vi "Z-Scan-20.vi"() -> ()   [LabVIEW 2014]
doc: "André Romero - 2020\nandretec@ifsc.usp.br"
uses:
  Z-Temporal-Signal.ctl
  <vilib>/Analysis/NI_AALBase.lvlib
panel:
  out "standard deviation":dbl format="%0.6f"
  out "ti/tf mean":dbl format="%0.2f"
  out "ti/tf Signal":dbl(graph)
  out "Number of samples":i32=4
  out "Time between acquire (ms)":u32=218
  out "Signal":dbl[][](graph)
  in  "rate":dbl=50000.0
  in  "N Samples":i64=8000
  out "Process time":string
  in  "Start Acquire":bool
  in  "Stop Acquire":bool
  out "Z Scan":cluster{"X":dbl, "Y":dbl}[](graph)
  # "DAQ Settings"
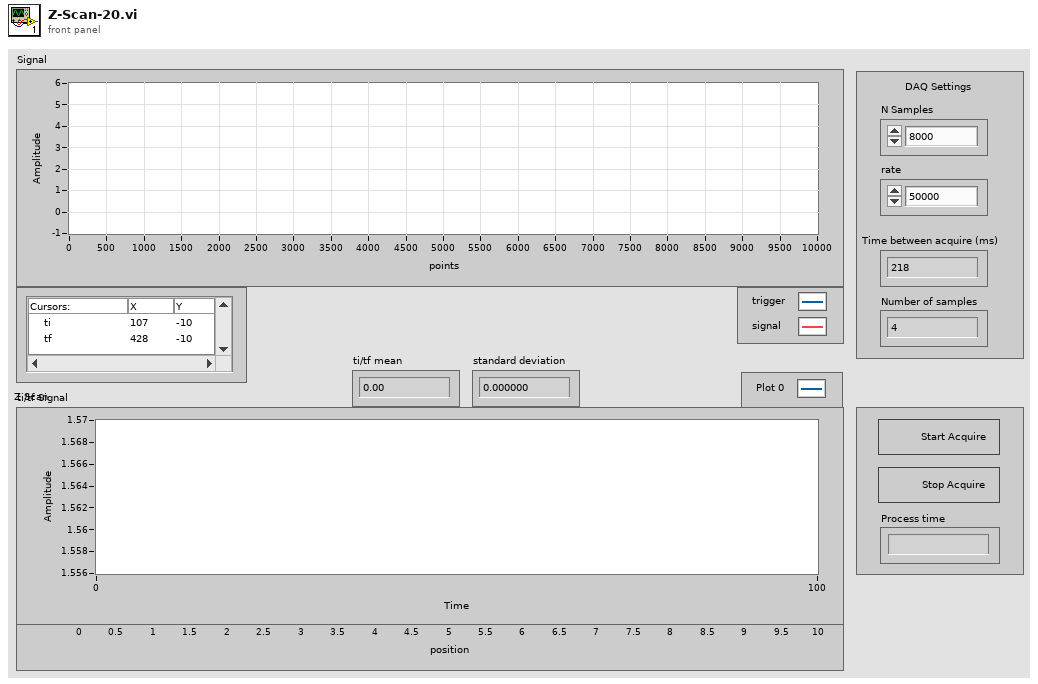
[diagram p1: front panel]
types:
  T1 = typedef "Z-Temporal-Signal.ctl" = cluster{"Signal State":string, "Signal":dbl[][], "ti":i32, "tf":i32, "Error":errorcluster}
  T2 = typedef "LVCursorListTypeDef.ctl" = cluster{"Name":string, "Color":u32, "Style":u8, "Point Style":u8, "Name Visible":bool, "Allow Drag":bool, "Cursor Mode":u32, "Plot":i32, "Index":i32, "Position":cluster{"X":dbl, "Y":dbl}, "X Scale":u32, "Y Scale":u32, "Watch Plots":i32[], "Watch All Plots":bool, "Plot Area":i32, "Label Offset":cluster{"X":dbl, "Y":dbl}}[]
  T3 = cluster{"Name":string, "Color":u32, "Style":u8, "Point Style":u8, "Name Visible":bool, "Allow Drag":bool, "Cursor Mode":u32, "Plot":i32, "Index":i32, "Position":cluster{"X":dbl, "Y":dbl}, "X Scale":u32, "Y Scale":u32, "Watch Plots":i32[], "Watch All Plots":bool, "Plot Area":i32, "Label Offset":cluster{"X":dbl, "Y":dbl}}
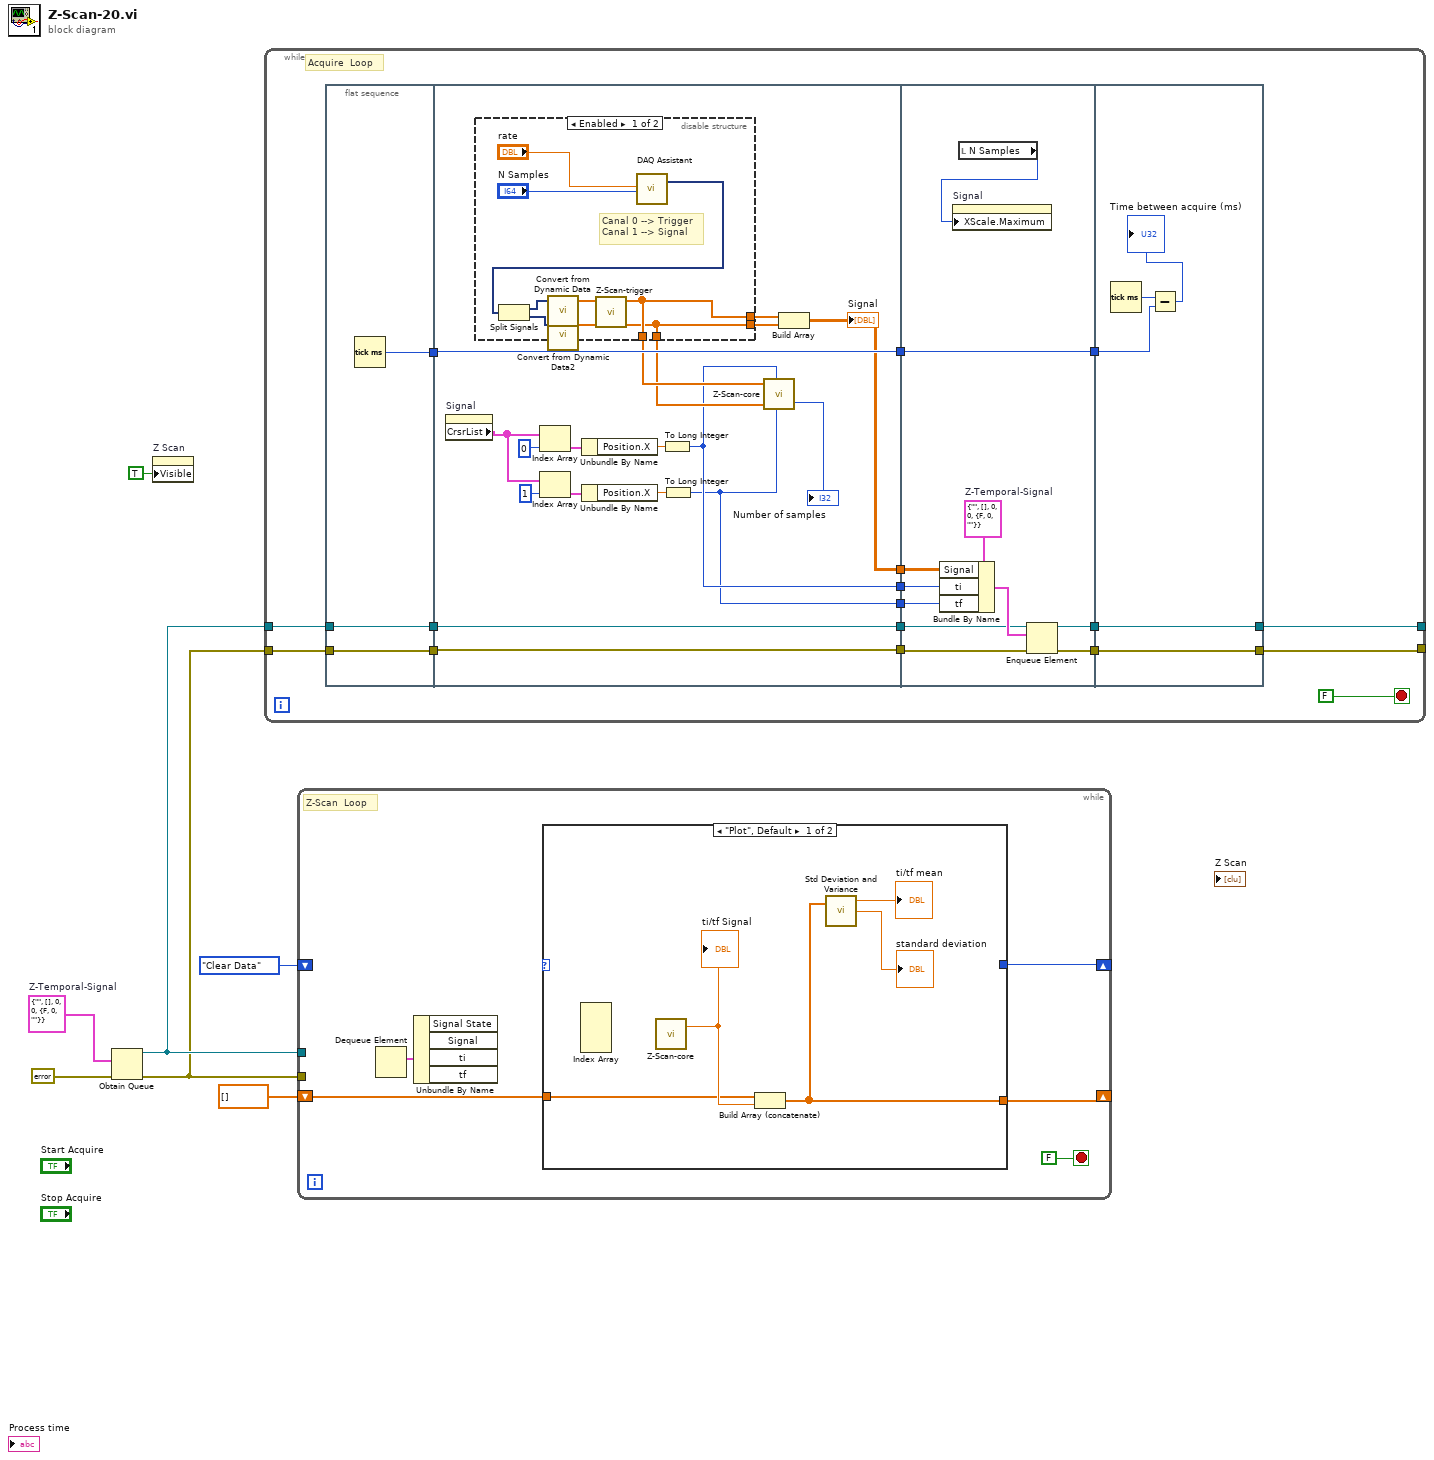
[diagram p0: block diagram]
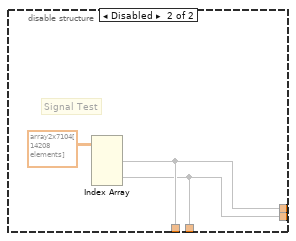
[diagram p2: hidden frame]
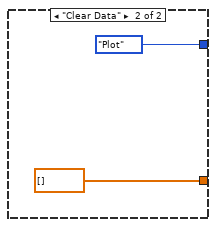
[diagram p3: hidden frame]
diagram:
  w4 = T1 {"Signal State"="", "Signal"=[], "ti"=0, "tf"=0, "Error"={"status"=FALSE, "code"=0, "source"=""}}  # Z-Temporal-Signal
  n1 = Obtain Queue(element data type=w4, error in (no error)=errorcluster {"status"=FALSE, "code"=0, "source"=""}) -> (queue out=w6:refnum<queue>, error out=w5:errorcluster)  [unwired: 3 in, 1 out]
  n2 = property on="Z Scan" class="XYGraph (strict)"("Visible"=TRUE) -> ()  [unwired: 2 in, 2 out]
  n3 = while {
    tunnel: w6 -> [w21]
    tunnel: w5 -> [w20]
    tunnel: [w18] -> _
    tunnel: [w8] -> _
    stop <- FALSE stop-if-true
    # "Acquire  Loop"
    n4 = flat-sequence {
      tunnel: [w27] -> w23
      tunnel: [w26] -> w22
      tunnel: w21 -> [w26]
      tunnel: w20 -> [w25]
      tunnel: [w25] -> w19
      tunnel: w23 -> [w43]
      tunnel: [w43] -> w17
      tunnel: w22 -> [w29]
      tunnel: w19 -> [w28]
      tunnel: [w32] -> w13
      tunnel: [w31] -> w12
      tunnel: [w30] -> w11
      tunnel: [w29] -> w10
      tunnel: [w28] -> w9
      tunnel: w17 -> [w68]
      tunnel: [w68] -> w16
      tunnel: [w65] -> w15
      tunnel: [w64] -> w14
      tunnel: w13 -> [w63]
      tunnel: w12 -> [w62]
      tunnel: w11 -> [w61]
      tunnel: w10 -> [w60]
      tunnel: w9 -> [w59]
      tunnel: w16 -> [w72]
      tunnel: [w70] -> w18
      tunnel: w15 -> [w70]
      tunnel: w14 -> [w69]
      tunnel: [w69] -> w8
      frame #0 {
        n5 = Tick Count (ms)() -> (millisecond timer value=w27:u32)
      }
      frame #1 {
        n6 = property on="Signal" class="WFGraph (strict)"() -> ("CrsrList"=w35:T2)  [unwired: 2 in, 2 out]
        n7 = disable-structure shown="Enabled" {
          disable-tunnel: [w47 w56] -> w45
          disable-tunnel: [w46 w55] -> w44
          disable-tunnel: [w47 w56] -> w34
          disable-tunnel: [w46 w55] -> w33
          frame Enabled {
            # "Canal 0 --> Trigger\nCanal 1 --> Signal"
            n8 = call "DAQ Assistant"("rate"="rate", "number of samples"="N Samples") -> ("data"=w52:dynamicdata)  [unwired: 15 in, 2 out]
            n9 = Split Signals(w52) -> (w51:dynamicdata, w50:dynamicdata)  [unwired: 2 in]
            n10 = call "Convert from Dynamic Data"("Dynamic Data Type"=w51) -> ("Array"=w49:dbl[])  [unwired: 3 in]
            n11 = call "Convert from Dynamic Data2"("Dynamic Data Type"=w50) -> ("Array"=w48:dbl[])  [unwired: 3 in]
            n12 = call "Z-Scan-trigger.vi"("signal in"=w48, "trigger in"=w49) -> ("signal out"=w46:dbl[], "trigger out"=w47:dbl[])  [unwired: 5 in, 1 out]
          }
          frame Disabled {
            # "Signal Test"
            n13 = Index Array(array=dbl[][] array2x7104[14208 elements] ("Signal 2")) -> (element #1=w56:dbl[], element #2=w55:dbl[])  [unwired: 4 in]
          }
        }
        n14 = Index Array(array=w35, index=0) -> (element=w38:T3)
        n15 = Index Array(array=w35, index=1) -> (element=w39:T3)
        n16 = Unbundle By Name(w38) -> ("Position.X"=w40:dbl)
        n17 = Unbundle By Name(w39) -> ("Position.X"=w41:dbl)
        n18 = To Long Integer(number=w40) -> (32bit integer=w31:i32)
        n19 = To Long Integer(number=w41) -> (32bit integer=w30:i32)
        n20 = call "Z-Scan-core.vi"("trigger in"=w34, "ti"=w31, "signal in"=w33, "tf"=w30) -> ("number of samples"=→"Number of samples":i32)  [unwired: 1 in, 1 out]
        n21 = Build Array(w45, w44) -> (w32:dbl[][])
        "Signal" <- w32
      }
      frame #2 {
        w67 = T1 {"Signal State"="", "Signal"=[], "ti"=0, "tf"=0, "Error"={"status"=FALSE, "code"=0, "source"=""}}  # Z-Temporal-Signal
        n22 = Bundle By Name(cluster=w67, "Signal"=w63, "ti"=w62, "tf"=w61) -> (w66:T1)
        n23 = local read "N Samples"() -> (w58:i64)
        n24 = property on="Signal" class="WFGraph (strict)"("XScale.Maximum"=w58) -> ()  [unwired: 2 in, 2 out]
        n25 = Enqueue Element(queue=w60, element=w66, error in (no error)=w59) -> (queue out=w65:refnum<queue>, error out=w64:errorcluster)  [unwired: 1 in, 1 out]
      }
      frame #3 {
        n26 = Tick Count (ms)() -> (millisecond timer value=w73:u32)
        n27 = Subtract(x=w73, y=w72) -> (x-y=→"Time between acquire (ms)":u32)
      }
    }
  }
  n28 = while {
    tunnel: w6 -> [_]
    tunnel: w5 -> [_]
    shift-right: [w76] -> _
    shift-left: dbl[] [] -> [w77]
    shift-right: [w75] -> _
    shift-left: enum16{"Clear Data", "Plot"}."Clear Data" -> [_]
    stop <- FALSE stop-if-true
    # "Z-Scan  Loop"
    n29 = Dequeue Element() -> (element=w74:T1)  [unwired: 3 in, 3 out]
    n30 = Unbundle By Name(w74) -> ()  [unwired: 4 out]
    n31 = case shown="\"Plot\", Default" {
      selector: _ -> [_ _]
      tunnel: w77 -> [w80 _]
      tunnel: [w79 dbl[] []] -> w76
      tunnel: [_ enum16{"Clear Data", "Plot"}."Plot"] -> w75
      frame "Plot", Default {
        n32 = Index Array() -> ()  [unwired: 5 in, 2 out]
        n33 = call "Z-Scan-core.vi"() -> ("mean tf/ti"=w83:dbl)  [unwired: 5 in, 1 out]
        "ti/tf Signal" <- w83
        n34 = Build Array (concatenate)(w80, w83) -> (w79:dbl[])
        n35 = call <vilib>:"Std Deviation and Variance.vi"("X"=w79) -> ("mean"=→"ti/tf mean":dbl, "standard deviation"=→"standard deviation":dbl)  [unwired: 1 in, 1 out]
      }
      frame "Clear Data" {
      }
    }
  }
